vi "SRV_Queue Streaming Restore States.vi"(8 "error in (no error)":errorcluster, 10 "Cached Streaming States":T1, 11 "Control Queue":refnum<queue>) -> (0 "error out":errorcluster, 3 "Control Queue out":refnum<queue>)   [LabVIEW 2014]
uses:
  Support/SRV_Command-Data Queue Data Type.ctl
  SRV_Streaming States.ctl
  SRV_Streaming State.ctl
  SRV_Streaming Modes.ctl
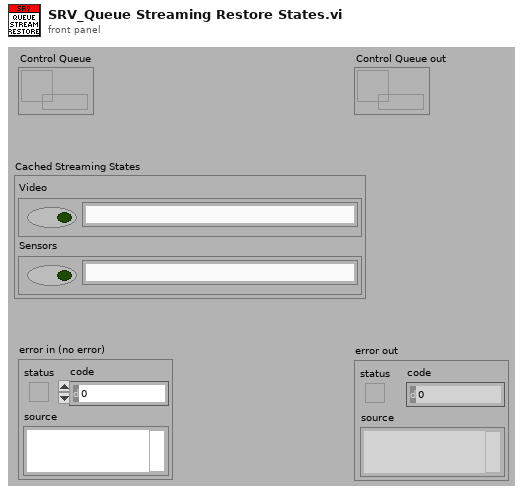
[diagram p1: front panel]
types:
  T1 = typedef "SRV_Streaming States.ctl" = cluster{"Video":T2, "Sensors":T2}
  T2 = typedef "SRV_Streaming State.ctl" = cluster{"Enabled":bool, "Data":string}
  T3 = typedef "SRV_Streaming Modes.ctl" = enum16{"Video", "Sensors"}
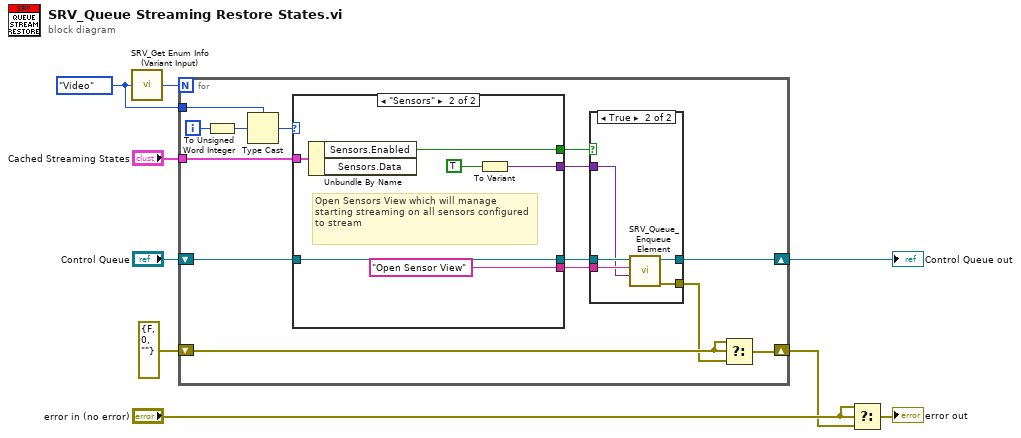
[diagram p0: block diagram]
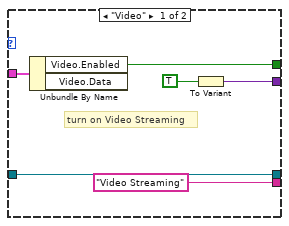
[diagram p2: hidden frame]
diagram:
  w6 = SRV_Streaming_Modes."Video" ("Streaming Modes")
  n1 = call "SRV_Get Enum Info (Variant Input).vi"("Variant (Enum)"=w6) -> ("Enum Size"=w7:i32)  [unwired: 4 in, 2 out]
  n2 = for {
    N: w7 -> [_]
    shift-right: [w23] -> w5
    shift-left: "Control Queue" -> [w17]
    tunnel: w6 -> [w20]
    tunnel: "Cached Streaming States" -> [w18]
    shift-right: [w10] -> w4
    shift-left: errorcluster {"status"=FALSE, "code"=0, "source"=""} ("error out") -> [w12]
    i -> [w22]
    n3 = To Unsigned Word Integer(number=w22) -> (unsigned 16bit integer=w21:u16)
    n4 = Type Cast(type=w20, x=w21) -> (*(type *) &x=w19:T3)
    n5 = case shown="\"Sensors\"" w19 {
      tunnel: w18 -> [w29 w35]
      tunnel: w17 -> [w28 w34]
      tunnel: [w28 w34] -> w16
      tunnel: [w27 w33] -> w15
      tunnel: ["Video Streaming" ("Command") "Open Sensor View" ("Command")] -> w14
      tunnel: [w25 w31] -> w13
      frame "Video" {
        # "turn on Video Streaming"
        n6 = Unbundle By Name(w29) -> ("Video.Enabled"=w27:bool)  [unwired: 1 out]
        n7 = To Variant(anything=TRUE ("Show Image")) -> (Variant=w25:variant)
      }
      frame "Sensors" {
        # "Open Sensors View which will manage starting streaming on all sensors configured to stream"
        n8 = Unbundle By Name(w35) -> ("Sensors.Enabled"=w33:bool)  [unwired: 1 out]
        n9 = To Variant(anything=TRUE ("Show Image")) -> (Variant=w31:variant)
      }
    }
    n10 = case shown="True" w15 {
      tunnel: w16 -> [w36 w41]
      tunnel: [w36 w40] -> w23
      tunnel: w14 -> [_ w39]
      tunnel: w13 -> [_ w38]
      tunnel: [_ w37] -> w11
      frame False {
      }
      frame True {
        n11 = call "SRV_Queue_Enqueue Element.vi"("Data"=w38, "Command"=w39, "Command-Data Queue"=w41) -> ("error out"=w37:errorcluster, "Command-Data Queue out"=w40:refnum<queue>)  [unwired: 6 in, 1 out]
      }
    }
    n12 = Select(t=w12, s=w12, f=w11) -> (s? t:f=w10:errorcluster)
  }
  "Control Queue out" <- w5
  n13 = Select(t="error in (no error)", s="error in (no error)", f=w4) -> (s? t:f=→"error out":errorcluster)
